vi "Preload station.vi"(0 "configuration file path":path caption="配置文件的路径", 1 "Preload station msic inf":cluster{"生产信息":refnum<vi>, "项目名称":refnum<vi>}) -> ()   [LabVIEW 2018]
uses:
  Ctl.xio/Preload station msic ctl.ctl
  SubVIS.xio/DataSocket/DataSocket_Tags.ctl
  Ctl.xio/part type.ctl
  SubVIS.xio/Creat Write List VI's/DefCtrl/Station.ctl
  <vilib>/Utility/file.llb/Read From Spreadsheet File (string).vi
  SubVIS.xio/DataSocket/Read PLC Vars/Read Bool Var.vi
  SubVIS.xio/DataSocket/Read PLC Vars/Read U32 Var.vi
  SubVIS.xio/DataSocket/Write PLC Vars/Write Bool Var in.vi
panel:
  in  "SQL information":string
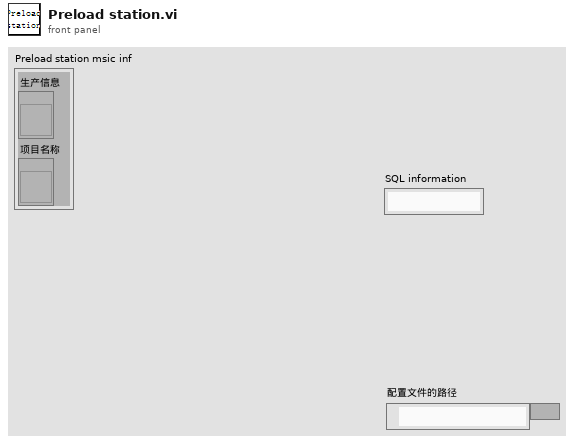
[diagram p1: front panel]
types:
  T1 = typedef "Station.ctl" = enum16{"粗切工位", "热处理工位", "精切工位", "PDF焊接工位", "打凹点预载力工位", "收卷工位", "EOL工位"}
  T2 = typedef "Preload station msic ctl.ctl" = cluster{"configuration file path":path, "DsOut":T3[], "Hopper car information":cluster{"Hopper car code":string, "Hopper car No":string, "plate No":string}, "pallet.produced number":i32, "SQL information":string, "Serial number":i32, "database path":path, "Preload station msic inf":cluster{"生产信息":refnum<vi>, "项目名称":refnum<vi>}, "part type":T4, "BarCode":string, "scanner resource name out":refnum<visa-resource-name>, "scanner coms":string}
  T3 = typedef "DataSocket_Tags.ctl" = cluster{"Ds ID":refnum<k13>, "Tag":string}
  T4 = typedef "part type.ctl" = cluster{"Part type":string, "Material code":string, "Part number":string, "Supplier code":string, "Line code":string, "Customer code":string, "Color code":string, "Upper limit":i32, "Temperature":string, "Tot time":string, "EOL stations":string}
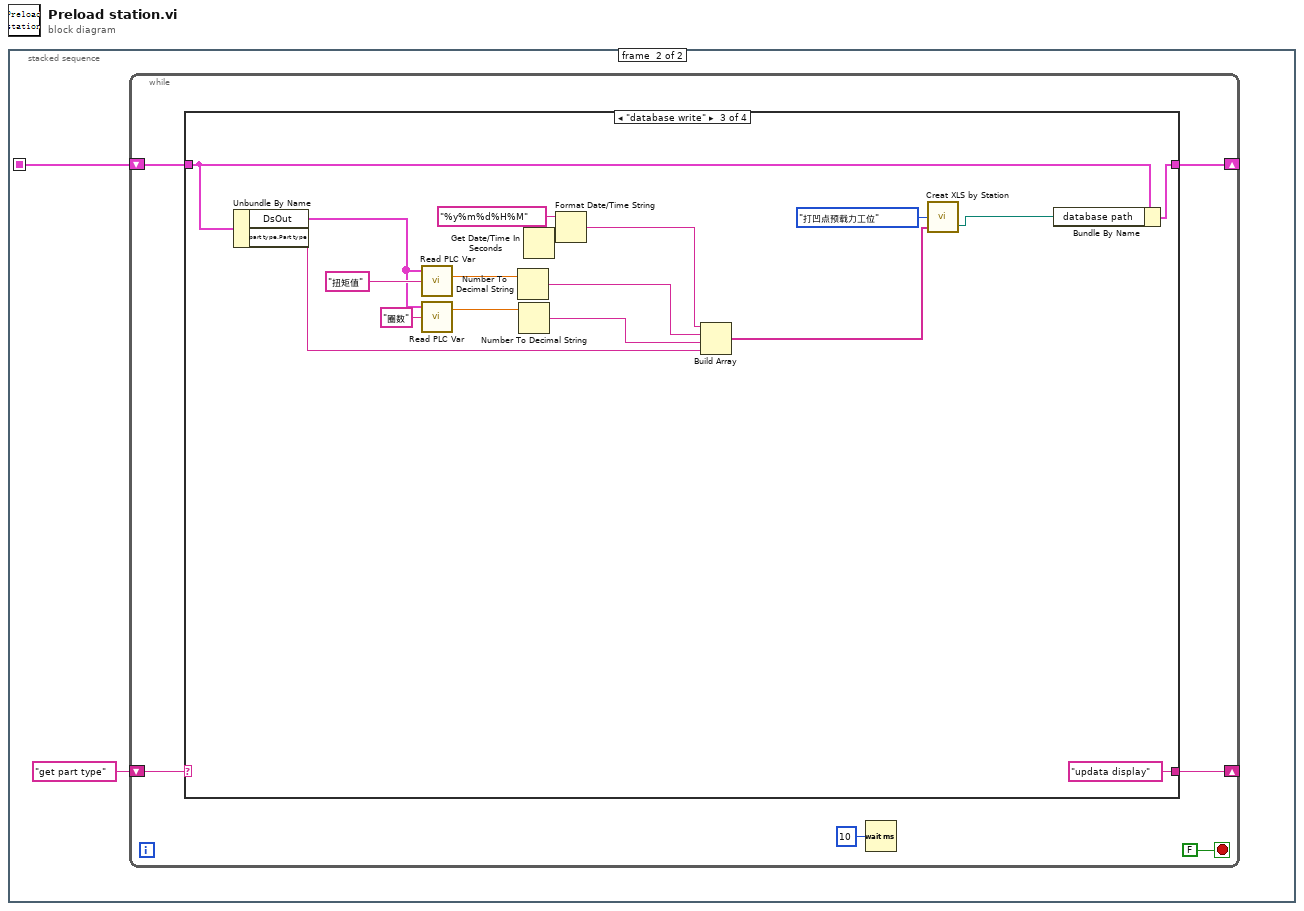
[diagram p0: block diagram]
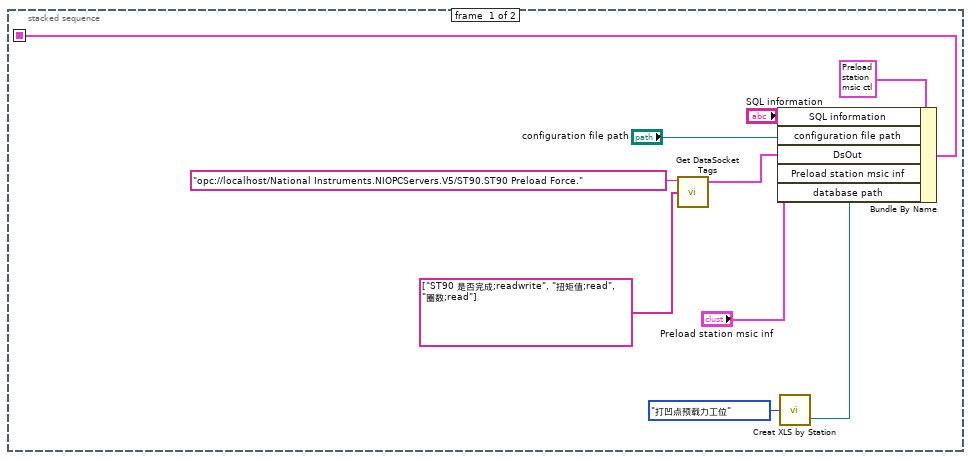
[diagram p2: hidden frame]
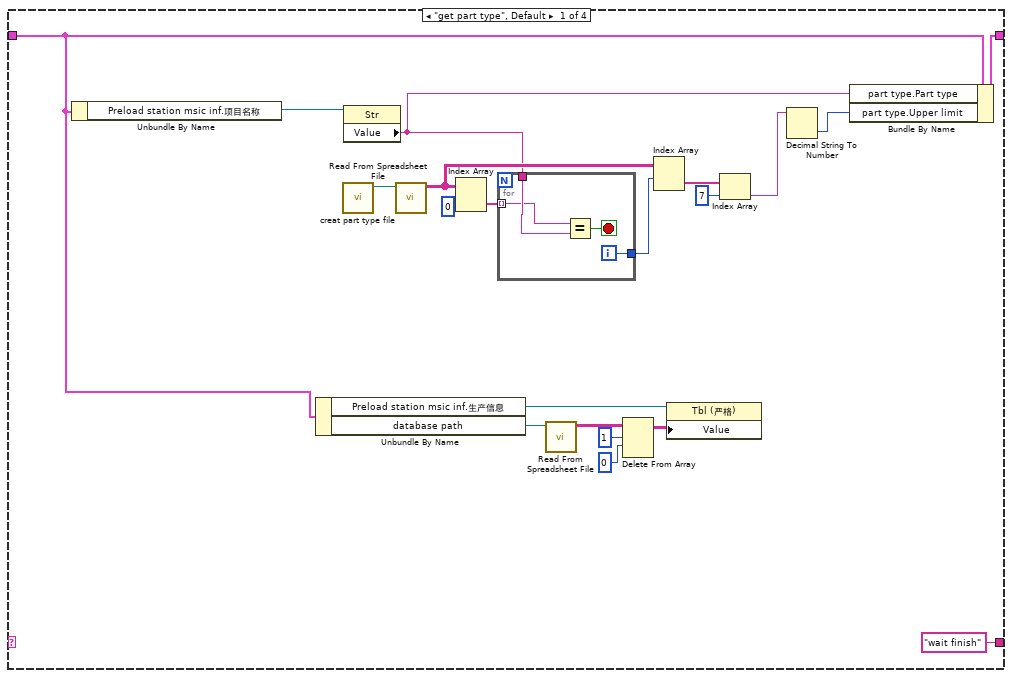
[diagram p3: hidden frame]
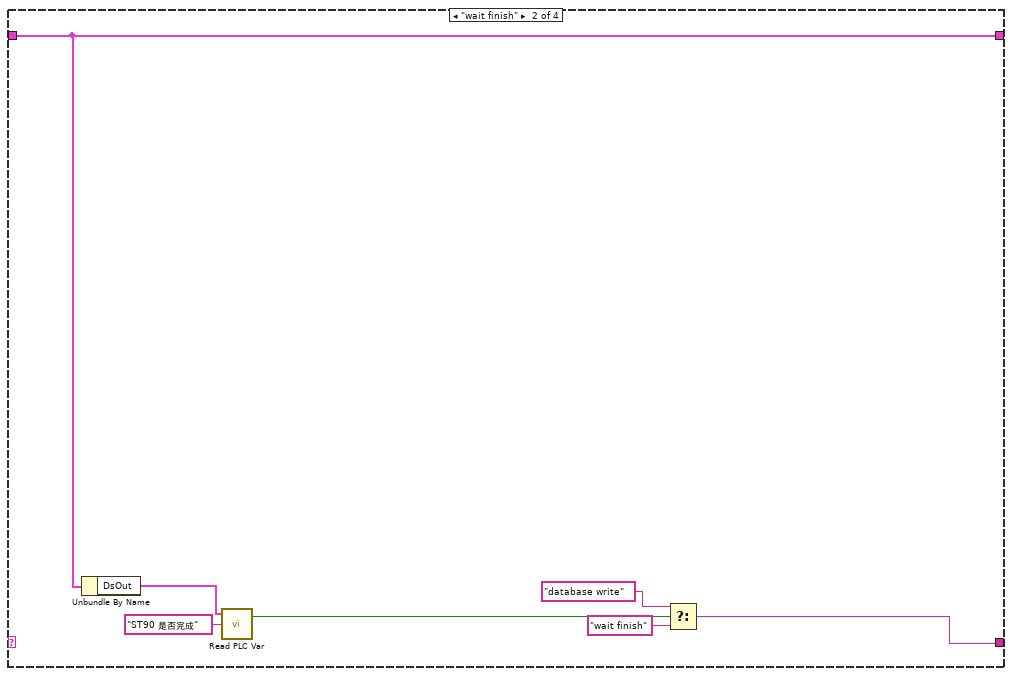
[diagram p4: hidden frame]
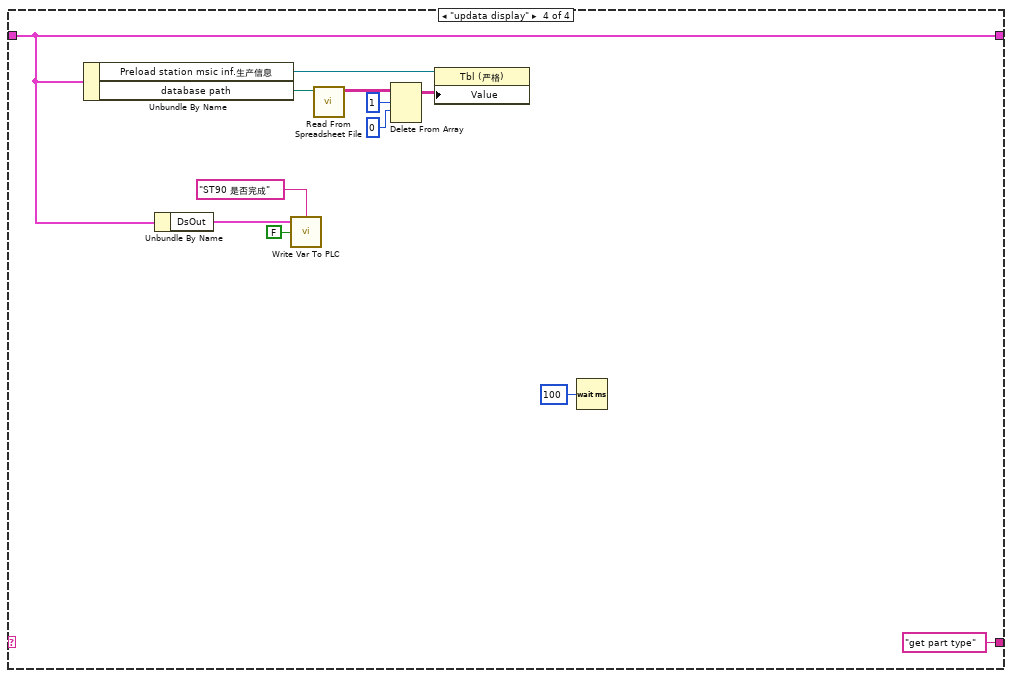
[diagram p5: hidden frame]
diagram:
  n1 = stacked-sequence {
    seq-local: [w6 _] -> [_ w12]
    frame #0 {
      n2 = call "Get DataSocket Tags.vi"("All Tags"=string[] ["ST90 是否完成;readwrite", "扭矩值;read", "圈数;read"], "URL"="opc://localhost/National Instruments.NIOPCServers.V5/ST90.ST90 Preload Force.") -> ("DsOut"=w10:T3[])  [unwired: 3 in]
      n3 = call "Creat XLS by Station.vi"("staiton"=Station."打凹点预载力工位") -> ("new file path (Not A Path if cancelled)"=w2:path)  [unwired: 5 in]
      n4 = Bundle By Name(cluster=T2 {"configuration file path"=path "", "DsOut"=[], "Hopper car information"={"Hopper car code"="", "Hopper car No"="", "plate No"=""}, "pallet.produced number"=0, "SQL information"="", "Serial number"=0, "database path"=path "", "Preload station msic inf"={"生产信息"=refnum, "项目名称"=refnum}, "part type"={"Part type"="", "Material code"="", "Part number"="", "Supplier code"="", "Line code"="", "Customer code"="", "Color code"="", "Upper limit"=0, "Temperature"="", "Tot time"="", "EOL stations"=""}, "BarCode"="", "scanner resource name out"="", "scanner coms"=""} ("PDF Welding msic ctl"), "SQL information"="SQL information", "configuration file path"="configuration file path", "DsOut"=w10, "Preload station msic inf"="Preload station msic inf", "database path"=w2) -> (w6:T2)
    }
    frame #1 {
      n5 = while {
        shift-right: [w18] -> _
        shift-left: w12 -> [w14]
        shift-right: [w17] -> _
        shift-left: "get part type" ("event") -> [w13]
        stop <- FALSE stop-if-true
        n6 = case shown="\"database write\"" w13 {
          tunnel: w14 -> [w19 w49 w64 w71]
          tunnel: [w37 w49 w65 w71] -> w18
          tunnel: ["wait finish" ("f") w44 "updata display" ("f") "get part type" ("f")] -> w17
          frame "get part type", Default {
            n7 = Unbundle By Name(w19) -> ("Preload station msic inf.项目名称"=w38:refnum<vi>)
            n8 = Unbundle By Name(w19) -> ("Preload station msic inf.生产信息"=w25:refnum<vi>, "database path"=w24:path)
            n9 = call "creat part type file.vi"() -> ("new file path (Not A Path if cancelled)"=w28:path)  [unwired: 11 in]
            n10 = property class="Str"(reference=w38) -> ("Value"=w27:string)  [unwired: 1 in, 2 out]
            n11 = call-poly <vilib>:"Read From Spreadsheet File.vi"("file path (dialog if empty)"=w28) -> ("all rows"=w33:string[][])  [unwired: 6 in, 4 out]
            n12 = Index Array(array=w33, index (col)=0 ("禁用的索引 (列)")) -> (element=w35:string[])  [unwired: 1 in]
            n13 = for {
              tunnel: w35 -> [w39] mode=indexing
              tunnel: [w41] -> w32
              tunnel: w27 -> [w40]
              i -> [w41]
              stop <- w42 stop-if-true
              n14 = Equal?(x=w39, y=w40) -> (x = y?=w42:bool)
            }
            n15 = call-poly <vilib>:"Read From Spreadsheet File.vi"("file path (dialog if empty)"=w24) -> ("all rows"=w23:string[][])  [unwired: 6 in, 4 out]
            n16 = Delete From Array(array=w23, length=1 ("长度"), index (row)=0 ("索引 (行)")) -> (array with subset deleted=w20:string[][])  [unwired: 1 in, 1 out]
            n17 = Index Array(array=w33, index (row)=w32) -> (element=w31:string[])  [unwired: 1 in]
            n18 = property class="Tbl (严格)"(reference=w25, "Value"=w20) -> ()  [unwired: 1 in, 2 out]
            n19 = Index Array(array=w31, index=7 ("索引")) -> (element=w30:string)
            n20 = Decimal String To Number(string=w30) -> (number=w29:i32)  [unwired: 2 in, 1 out]
            n21 = Bundle By Name(cluster=w19, "part type.Part type"=w27, "part type.Upper limit"=w29) -> (w37:T2)
          }
          frame "wait finish" {
            n22 = Unbundle By Name(w49) -> ("DsOut"=w48:T3[])
            n23 = call-poly "Read PLC Var.vi"("Tag IN"="ST90 是否完成", "Ds PLCTags IN"=w48) -> ("Bool Var out"=w46:bool)  [unwired: 1 in, 1 out]
            n24 = Select(t="database write" ("f"), s=w46, f="wait finish") -> (s? t:f=w44:string)
          }
          frame "database write" {
            n25 = Unbundle By Name(w64) -> ("DsOut"=w62:T3[], "part type.Part type"=w53:string)
            n26 = call-poly "Read PLC Var.vi"("Tag IN"="扭矩值", "Ds PLCTags IN"=w62) -> ("U32 Var out"=w60:dbl)  [unwired: 1 in, 1 out]
            n27 = call-poly "Read PLC Var.vi"("Tag IN"="圈数", "Ds PLCTags IN"=w62) -> ("U32 Var out"=w59:dbl)  [unwired: 1 in, 1 out]
            n28 = Number To Decimal String(number=w60) -> (decimal integer string=w58:string)  [unwired: 1 in]
            n29 = Number To Decimal String(number=w59) -> (decimal integer string=w57:string)  [unwired: 1 in]
            n30 = Get Date/Time In Seconds() -> (seconds since 1Jan1904=w56:timestamp)
            n31 = Format Date/Time String(time format string (%c)="%y%m%d%H%M" ("时间格式字符串(%c)"), seconds (now)=w56) -> (date/time string=w54:string)  [unwired: 1 in]
            n32 = Build Array(w54, w58, w57, w53) -> (w50:string[])
            n33 = call "Creat XLS by Station.vi"("staiton"=Station."打凹点预载力工位", "data in"=w50) -> ("new file path (Not A Path if cancelled)"=w51:path)  [unwired: 4 in]
            n34 = Bundle By Name(cluster=w64, "database path"=w51) -> (w65:T2)
          }
          frame "updata display" {
            n35 = Unbundle By Name(w71) -> ("Preload station msic inf.生产信息"=w77:refnum<vi>, "database path"=w76:path)
            n36 = Unbundle By Name(w71) -> ("DsOut"=w70:T3[])
            n37 = call-poly "Write Var To PLC.vi"("Tag IN"="ST90 是否完成", "Bool Var in"=FALSE, "Ds PLCTags IN"=w70) -> ()  [unwired: 1 in, 2 out]
            n38 = call-poly <vilib>:"Read From Spreadsheet File.vi"("file path (dialog if empty)"=w76) -> ("all rows"=w75:string[][])  [unwired: 6 in, 4 out]
            n39 = Delete From Array(array=w75, length=1 ("长度"), index (row)=0 ("索引 (行)")) -> (array with subset deleted=w72:string[][])  [unwired: 1 in, 1 out]
            n40 = property class="Tbl (严格)"(reference=w77, "Value"=w72) -> ()  [unwired: 1 in, 2 out]
            n41 = Wait (ms)(milliseconds to wait=u32 100 ("等待时间（毫秒）")) -> ()  [unwired: 1 out]
          }
        }
        n42 = Wait (ms)(milliseconds to wait=u32 10 ("等待时间（毫秒）")) -> ()  [unwired: 1 out]
      }
    }
  }
